vi "Servo Set Pulse Width.vi"(8 "Error In":errorcluster, 9 "Pulse Widths (uS)":u16[](array[numeric]), 10 "Channels":u8[](array[numeric]), 11 "LINX Device Config":T1) -> (0 "Error Out":errorcluster, 3 "LINX Device Config":T1)   [LabVIEW 2014, in "LMH-LINX.lvlib" / "Device.lvlib"]
uses:
  Device.lvlib
  Type Defs/LINX Device Config.ctl
  Type Defs/Interface.ctl
  Type Defs/TCP Config.ctl
  Type Defs/Channels.ctl
  Type Defs/Error Type.ctl
  LMH-LINX.lvlib
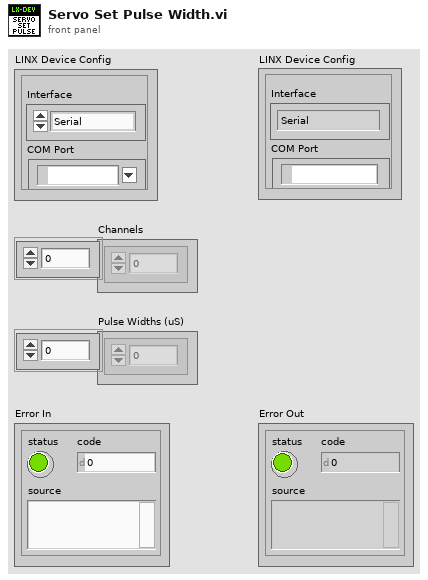
[diagram p1: front panel]
types:
  T1 = typedef "LMH-LINX.lvlib/Device.lvlib/LINX Device Config.ctl" = cluster{"Interface":T2, "COM Port":refnum<visa-resource-name>, "TCP Configuration":T3, "Device Family":u8, "Device ID":u8, "Device Name":string, "TCP Ref":refnum<k5>, "Channels":T4}
  T2 = typedef "LMH-LINX.lvlib/Interface.ctl" = enum16{"Serial", "TCP"}
  T3 = typedef "LMH-LINX.lvlib/Device.lvlib/TCP Config.ctl" = cluster{"IP Address":string, "Port":u16}
  T4 = typedef "LMH-LINX.lvlib/Channels.ctl" = cluster{"DI":u8[], "DO":u8[], "AI":u8[], "AO":u8[], "PWM":u8[], "QE":u8[], "UART":u8[], "I2C 2":u8[], "SPI":u8[], "CAN":u8[], "Servo":u8[], "AI Ref (V)":dbl, "AI Resolution (Bits)":u8, "AO Ref (V)":dbl, "AO Resolution (Bits)":u8}
  T5 = typedef "LMH-LINX.lvlib/Error Type.ctl" = enum16{"Unknown", "Timeout", "Corrupt Return Packet", "Unable To Connect", "Command Not Supported", "Channel DNE", "Invalid COM Config", "Firmware Version Mismatch", "myRIO Support", "CMD Specific Error", "Local IO Not Supported"}
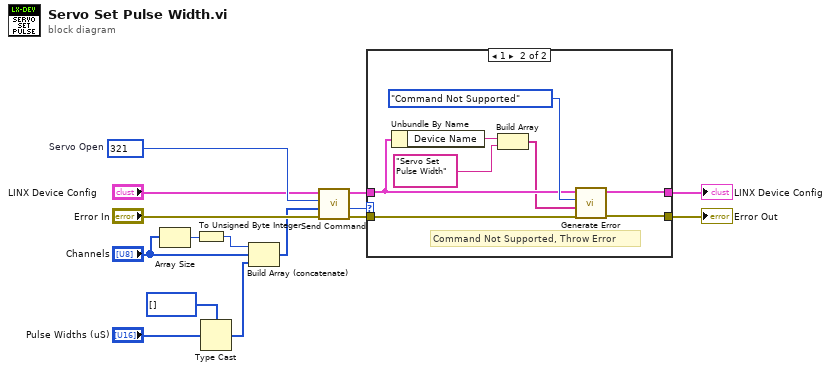
[diagram p0: block diagram]
diagram:
  w14 = u16 321  # Servo Open
  n1 = Array Size(array="Channels") -> (size(s)=w3:i32)
  n2 = To Unsigned Byte Integer(number=w3) -> (unsigned 8bit integer=w1:u8)
  n3 = Type Cast(type=u8[] [] ("Channels"), x="Pulse Widths (uS)") -> (*(type *) &x=w4:u8[])
  n4 = Build Array (concatenate)(w1, "Channels", w4) -> (w5:u8[])
  n5 = call "Send Command.vi"("Error In"="Error In", "ARGS"=w5, "CMD"=w14, "LINX Device Config"="LINX Device Config") -> ("Error Out"=w9:errorcluster, "Status"=w8:u8, "LINX Device Config"=w11:T1)  [unwired: 4 in, 1 out]
  n6 = case shown="1" w8 {
    tunnel: [w17 w23] -> w12
    tunnel: w11 -> [w17 w19]
    tunnel: [w16 w24] -> w10
    tunnel: w9 -> [w16 w25]
    frame 0, Default {
      # "Status OK, Process Data"
    }
    frame 1 {
      # "Command Not Supported, Throw Error"
      n7 = Unbundle By Name(w19) -> ("Device Name"=w21:string)
      n8 = Build Array(w21, "Servo Set Pulse Width") -> (w18:string[])
      n9 = call "Generate Error.vi"("Error In"=w25, "Arguments"=w18, "Error Type"=Error_Type."Command Not Supported", "LINX Device Config"=w19) -> ("Error Out"=w24:errorcluster, "Dup LINX Device Config"=w23:T1)  [unwired: 6 in]
    }
  }
  "Error Out" <- w10
  "LINX Device Config" <- w12
